vi "QuadrantToSigns.vi"(0 "Point":cluster{"X":sgl, "Y":sgl, "Z":sgl}={"X"=1.0, "Y"=1.0, "Z"=1.0}, 1 "Quadrant":i32) -> (14 "Point Out":cluster{"X":sgl, "Y":sgl, "Z":sgl})   [LabVIEW 2014]
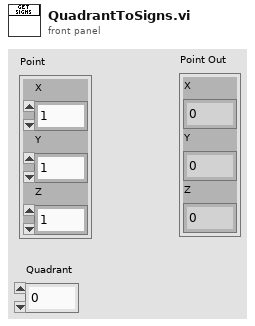
[diagram p1: front panel]
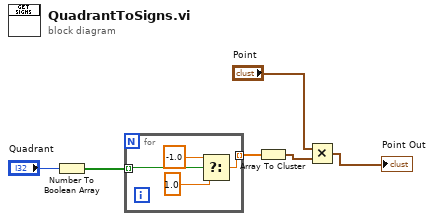
[diagram p0: block diagram]
diagram:
  n1 = Number To Boolean Array(number="Quadrant") -> (Boolean array=w5:bool[])
  n2 = for {
    tunnel: w5 -> [w10] mode=indexing
    tunnel: [w7] -> w4 mode=indexing
    n3 = Select(t=-1.0, s=w10, f=1.0) -> (s? t:f=w7:dbl)
  }
  n4 = Array To Cluster(array=w4) -> (cluster=w3:cluster{"[0]":dbl, "[1]":dbl, "[2]":dbl})
  n5 = Multiply(x="Point", y=w3) -> (x*y=→"Point Out":cluster{dbl, dbl, dbl})
